vi "Get Worker Count.vi"(8 "error in (no error)":errorcluster, 11 "Comm Interface in":refnum<class "Comm Interface.lvclass">) -> (0 "error out":errorcluster, 2 "Worker Count":i32, 3 "Comm Interface out":refnum<class "Comm Interface.lvclass">)   [LabVIEW 2017, in "Comm Interface.lvlib" / "Comm Interface.lvclass"]
uses:
  Comm Interface.lvclass
  Comm Interface.lvclass/Comm Interface.ctl
  WebSocket Server/Actors/Connection Listener/Connection Listener Messages/Get Connection List Msg/Get Connection List Msg.lvclass
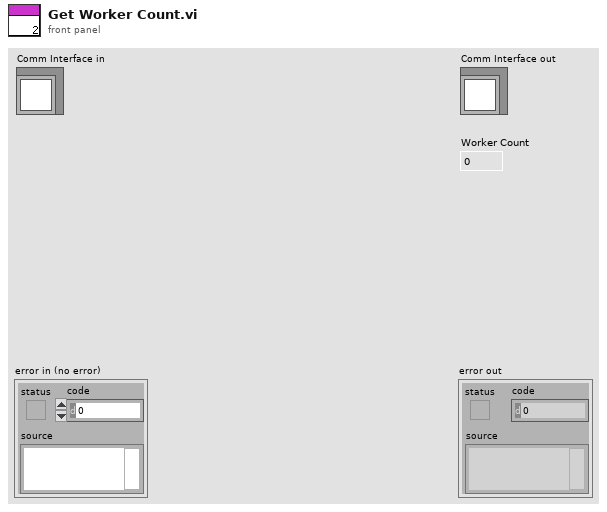
[diagram p1: front panel]
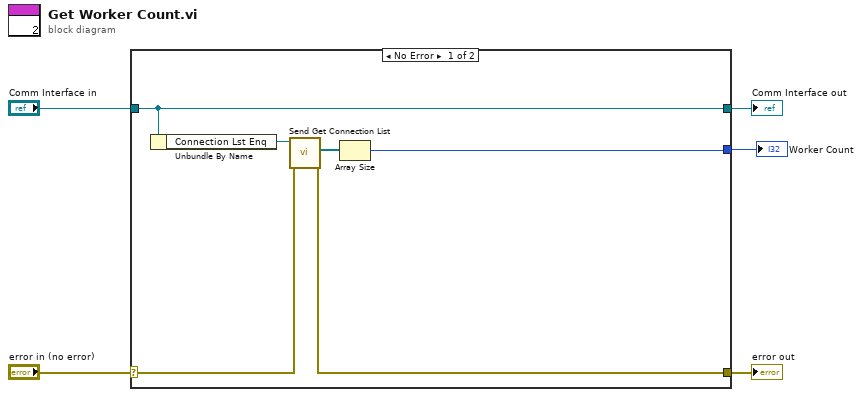
[diagram p0: block diagram]
diagram:
  n1 = case shown="No Error" "error in (no error)" {
    selector: "error in (no error)" -> [w9 w13]
    tunnel: [w8 w13] -> w4
    tunnel: [w11 w12] -> w2
    tunnel: "Comm Interface in" -> [w11 w12]
    tunnel: [w6 _] -> w1
    frame No Error {
      n2 = Unbundle By Name(w11) -> ("Connection Lst Enq"=w10:refnum<class "Message Enqueuer.lvclass">)
      n3 = call "Send Get Connection List.vi"("error in (no error)"=w9, "Message Enqueuer in"=w10) -> ("error out"=w8:errorcluster, "Connection List"=w7:refnum<class "Message Enqueuer.lvclass">[])  [unwired: 7 in, 1 out]
      n4 = Array Size(array=w7) -> (size(s)=w6:i32)
    }
    frame Error {
    }
  }
  "error out" <- w4
  "Comm Interface out" <- w2
  "Worker Count" <- w1
